vi "verbindungs_fehler.vi"() -> (0 "schließen?":bool)   [LabVIEW 2010]
panel:
  in  "Schließen":bool
  out "String":string="!!!Fehler bei verbindung zum Interface!!!\nÜberprüfen Sie bitte die Verbindung, dann klicken Sie auf Weiter.\nAndernfalls auf Schließen"
  in  "ende?":bool
  in  "weiter":bool
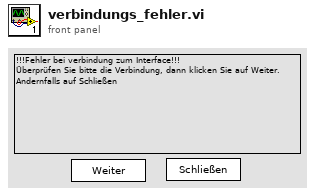
[diagram p1: front panel]
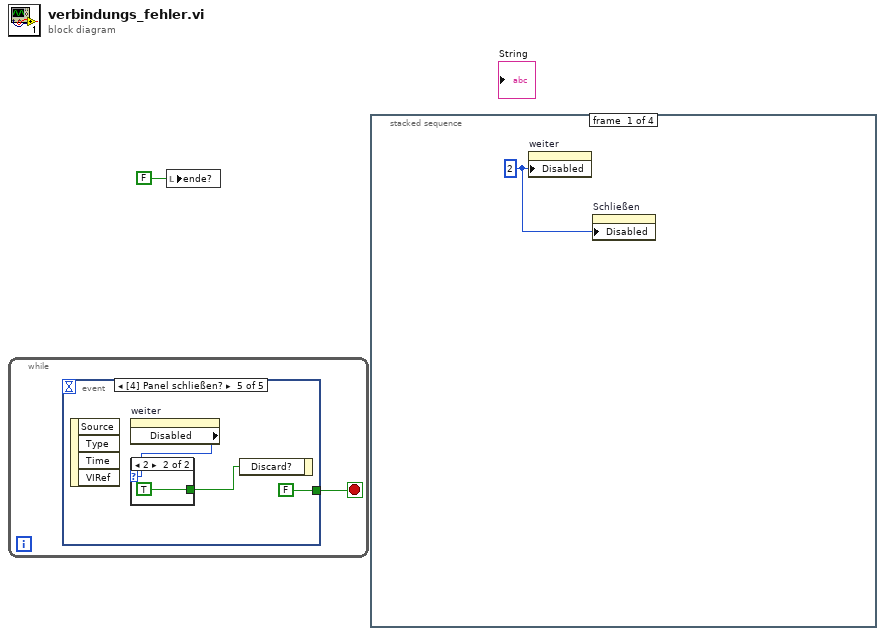
[diagram p0: block diagram]
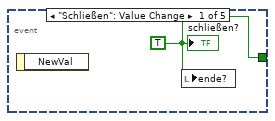
[diagram p2: hidden frame]
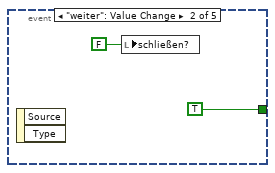
[diagram p3: hidden frame]
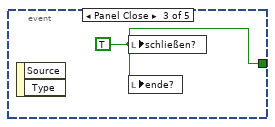
[diagram p4: hidden frame]
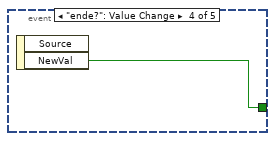
[diagram p5: hidden frame]
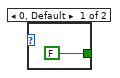
[diagram p6: hidden frame]
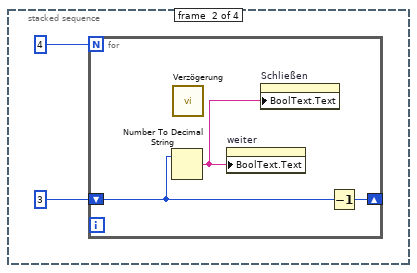
[diagram p7: hidden frame]
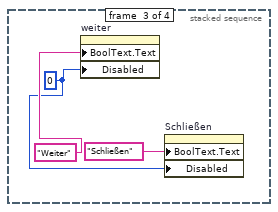
[diagram p8: hidden frame]
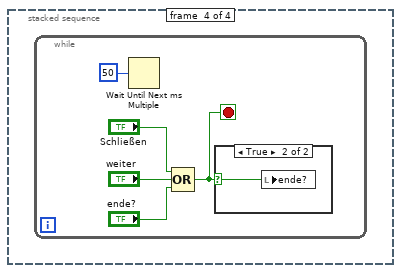
[diagram p9: hidden frame]
diagram:
  n1 = while {
    stop <- w2 stop-if-true
    n2 = event shown="[4] Panel schließen?" {
      selector: _ -> [_ _ _ _ _]
      dyn-events: _ -> [_ _ _ _ _]
      timeout: _ -> [_ _ _ _ _]
      tunnel: [w3 TRUE ("NewVal") w6 w7 FALSE ("NewVal")] -> w2
      event "Schließen": Value Change {
        w3 = TRUE ("schließen?")
        n3 = event-data() -> ()  [unwired: 2 out]
        n4 = local write "ende?"(w3) -> ()
        "schließen?" <- w3
      }
      event "weiter": Value Change {
        n5 = event-data() -> ()  [unwired: 3 out]
        n6 = local write "schließen?"(FALSE ("schließen?")) -> ()
      }
      event Panel Close {
        w6 = TRUE ("ende?")
        n7 = event-data() -> ()  [unwired: 3 out]
        n8 = local write "schließen?"(w6) -> ()
        n9 = local write "ende?"(w6) -> ()
      }
      event "ende?": Value Change {
        n10 = event-data() -> ("NewVal"=w7:bool)  [unwired: 2 out]
      }
      event Panel Close? {
        n11 = event-data() -> ()  [unwired: 5 out]
        n12 = property on="weiter" class="Bool."() -> ("Disabled"=w10:u8)  [unwired: 2 in, 2 out]
        n13 = case shown="2" w10 {
          tunnel: [FALSE TRUE] -> w9
          frame 0, Default {
          }
          frame 2 {
          }
        }
        n14 = event-data("Discard?"=w9) -> ()  [unwired: 1 in, 1 out]
      }
    }
  }
  n15 = local write "ende?"(FALSE ("ende?")) -> ()
  n16 = stacked-sequence {
    frame #0 {
      w13 = u8 2 ("Deaktiviert")
      n17 = property on="weiter" class="Bool."("Disabled"=w13) -> ()  [unwired: 2 in, 2 out]
      n18 = property on="Schließen" class="Bool."("Disabled"=w13) -> ()  [unwired: 2 in, 2 out]
    }
    frame #1 {
      n19 = for {
        N: 4 -> [_]
        shift-right: [w17] -> _
        shift-left: 3 -> [w18]
        n20 = Number To Decimal String(number=w18) -> (decimal integer string=w16:string)  [unwired: 1 out]
        n21 = call "Verzögerung"() -> ()  [unwired: 2 in, 10 out]
        n22 = property on="weiter" class="Bool."("BoolText.Text"=w16) -> ()  [unwired: 2 in, 2 out]
        n23 = property on="Schließen" class="Bool."("BoolText.Text"=w16) -> ()  [unwired: 2 in, 2 out]
        n24 = Decrement(x=w18) -> (x-1=w17:i32)
      }
    }
    frame #2 {
      w19 = u8 0 ("Deaktiviert")
      n25 = property on="weiter" class="Bool."("BoolText.Text"="Weiter" ("Boolescher Text.Text"), "Disabled"=w19) -> ()  [unwired: 2 in, 2 out]
      n26 = property on="Schließen" class="Bool."("BoolText.Text"="Schließen" ("Boolescher Text.Text"), "Disabled"=w19) -> ()  [unwired: 2 in, 2 out]
    }
    frame #3 {
      n27 = while {
        stop <- w22 stop-if-true
        n28 = Wait Until Next ms Multiple(millisecond multiple=50) -> ()  [unwired: 1 out]
        n29 = Compound Arithmetic op=OR("Schließen", "weiter", "ende?") -> (w22:bool)
        n30 = case shown="True" w22 {
          selector: w22 -> [_ w27]
          frame False {
          }
          frame True {
            n31 = local write "ende?"(w27) -> ()
          }
        }
      }
    }
  }
